vi "Handle Parameter Configuration File Change.vi"(8 "error in":errorcluster, 10 "new parameter configuration file path":path, 11 "Ballard MIL-STD-1553 custom device in":T1 format="%.0x") -> (0 "error out":errorcluster, 2 "parameters configuration file out":path, 3 "Ballard MIL-STD-1553 custom device out":T1 format="%.0x")   [LabVIEW 2020, in "Ballard MIL-STD-1553 System Explorer.lvlib" / "Implementation.lvlib" / "Refresh.lvlib"]
uses:
  Refresh.lvlib
  Scripting/Ballard MIL-STD-1553 Scripting.lvlib
  Import/MIL-STD 1553 Import.lvlib
  <vilib>/NI VeriStand/Custom Device API/Custom Device Item Ref.ctl
  <vilib>/NI VeriStand/Custom Device API/Custom Device API.lvlib
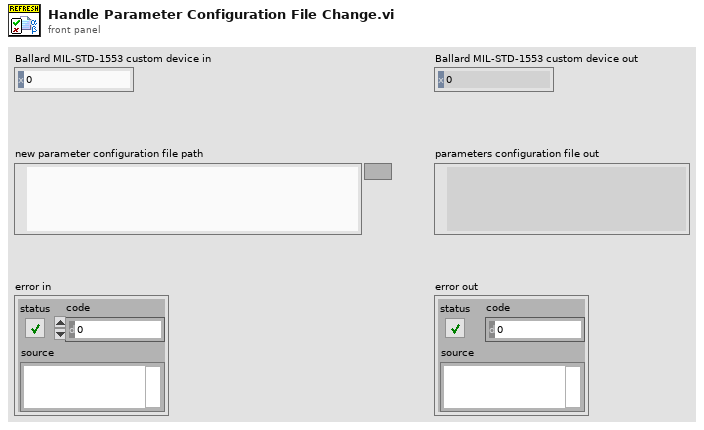
[diagram p1: front panel]
types:
  T1 = typedef "Custom Device API.lvlib/Custom Device Item Ref.ctl" = u64
  T2 = typedef "1553 Channel.ctl" = cluster{"HW channel":u16, "terminals":T3[], "messages":T5[], "acyclic frame names":string[]}
  T3 = typedef "Terminal Name and Address.ctl" = cluster{"name":string, "terminal address":T4}
  T4 = typedef "Address.ctl" = u16
  T5 = typedef "Message Definition.ctl" = cluster{"name":string, "message type":T6, "endpoint Rx":T7, "endpoint Tx":T7, "mode code":u16, "number of words":u16, "parameters":cluster{"name":string, "default value":dbl, "unit":string, "parameter definition":T8}[], "create timestamp channel":bool}
  T6 = typedef "Message Type.ctl" = string
  T7 = typedef "Terminal Endpoint.ctl" = cluster{"terminal address":T4, "subaddress":T4}
  T8 = typedef "Parameter Definition.ctl" = cluster{"start index":i32, "size (bits)":i32, "encoding":enum16{"BNR", "BCD", "Discrete"}, "signed":bool, "multiplier":dbl, "offset":dbl}
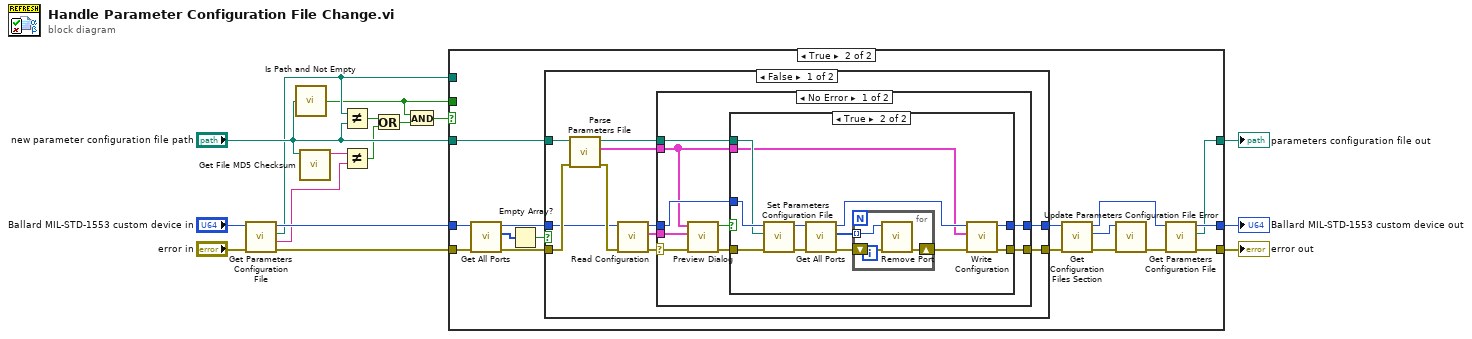
[diagram p0: block diagram]
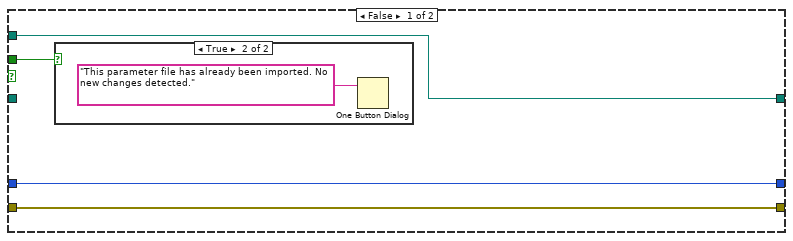
[diagram p2: hidden frame]
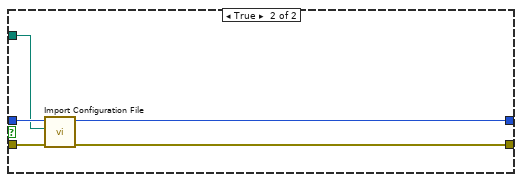
[diagram p6: hidden frame]
diagram:
  n1 = call "Get Parameters Configuration File.vi"("error in"="error in", "Ballard MIL-STD 1553 custom device in"="Ballard MIL-STD-1553 custom device in") -> ("error out"=w16:errorcluster, "MD5 checksum"=w8:string, "parameters configuration file"=w7:path, "Ballard MIL-STD 1553 custom device out"=w14:T1)  [unwired: 6 in]
  n2 = call <vilib>:"Is Path and Not Empty.vi"("path"="new parameter configuration file path") -> ("Is Path and Not Empty?"=w1:bool)  [unwired: 4 in]
  n3 = call "Get File MD5 Checksum.vi"("path"="new parameter configuration file path") -> ("MD5"=w4:string)  [unwired: 9 in, 1 out]
  n4 = Not Equal?(x=w7, y="new parameter configuration file path") -> (x != y?=w6:bool)
  n5 = Not Equal?(x=w4, y=w8) -> (x != y?=w5:bool)
  n6 = Or(x=w6, y=w5) -> (x .or. y?=w3:bool)
  n7 = And(x=w1, y=w3) -> (x .and. y?=w2:bool)
  n8 = case shown="True" w2 {
    tunnel: w16 -> [w19 w30]
    tunnel: w14 -> [w20 w31]
    tunnel: [w19 w25] -> w12
    tunnel: [w20 w23] -> w11
    tunnel: "new parameter configuration file path" -> [_ w32]
    tunnel: [w18 w22] -> w10
    tunnel: w7 -> [w18 _]
    tunnel: w1 -> [w17 _]
    frame False {
      n9 = case shown="True" w17 {
        frame False {
        }
        frame True {
          n10 = One Button Dialog(message="This parameter file has already been imported. No new changes detected.") -> ()  [unwired: 1 in, 1 out]
        }
      }
    }
    frame True {
      n11 = call "Get All Ports.vi"("error in"=w30, "Ballard MIL-STD 1553 custom device in"=w31) -> ("error out"=w29:errorcluster, "ports"=w27:T1[], "Ballard MIL-STD 1553 custom device out"=w28:T1)  [unwired: 7 in]
      n12 = Empty Array?(array=w27) -> (empty?=w26:bool)
      n13 = case shown="False" w26 {
        tunnel: [w40 w80] -> w35
        tunnel: [w38 w79] -> w34
        tunnel: w28 -> [w44 w78]
        tunnel: w29 -> [w46 w77]
        tunnel: w32 -> [w47 w76]
        frame False {
          n14 = call "Parse Parameters File.vi"("error in"=w46, "path to XML document"=w47) -> ("error out"=w45:errorcluster, "1553 channels"=w42:T2[], "path to XML document out"=w37:path)  [unwired: 7 in]
          n15 = call "Read Configuration.vi"("error in"=w45, "Ballard MIL-STD 1553 custom device in"=w44) -> ("error out"=w43:errorcluster, "1553 channels"=w41:T2[], "Ballard MIL-STD 1553 custom device out"=w39:T1)  [unwired: 7 in]
          n16 = case shown="No Error" w43 {
            selector: w43 -> [w55 w74]
            tunnel: w42 -> [w50 _]
            tunnel: w41 -> [w56 _]
            tunnel: [w49 w75] -> w40
            tunnel: w39 -> [w52 w75]
            tunnel: [w48 w74] -> w38
            tunnel: w37 -> [w51 _]
            frame No Error {
              n17 = call "Preview Dialog.vi"("error in"=w55, "current configuration"=w56, "new configuration"=w50) -> ("error out"=w53:errorcluster, "apply changes"=w54:bool)  [unwired: 7 in]
              n18 = case shown="True" w54 {
                tunnel: w53 -> [w57 w62]
                tunnel: w52 -> [w58 w64]
                tunnel: w51 -> [_ w63]
                tunnel: w50 -> [_ w61]
                tunnel: [w58 w60] -> w49
                tunnel: [w57 w59] -> w48
                frame False {
                }
                frame True {
                  n19 = call "Set Parameters Configuration File.vi"("error in"=w62, "parameters configuration file path"=w63, "Ballard MIL-STD 1553 custom device in"=w64) -> ("error out"=w69:errorcluster, "Ballard MIL-STD 1553 custom device out"=w70:T1)  [unwired: 7 in]
                  n20 = call "Get All Ports.vi"("error in"=w69, "Ballard MIL-STD 1553 custom device in"=w70) -> ("error out"=w68:errorcluster, "ports"=w65:T1[], "Ballard MIL-STD 1553 custom device out"=w66:T1)  [unwired: 7 in]
                  n21 = for {
                    shift-right: [w72] -> w67
                    shift-left: w68 -> [w73]
                    tunnel: w65 -> [w71] mode=indexing
                    n22 = call "Remove Port.vi"("error in"=w73, "port"=w71) -> ("error out"=w72:errorcluster)  [unwired: 9 in]
                  }
                  n23 = call "Write Configuration.vi"("error in"=w67, "1553 channels"=w61, "Ballard MIL-STD 1553 custom device in"=w66) -> ("error out"=w59:errorcluster, "Ballard MIL-STD 1553 custom device out"=w60:T1)  [unwired: 7 in]
                }
              }
            }
            frame Error {
            }
          }
        }
        frame True {
          n24 = call "Import Configuration File.vi"("error in"=w77, "parameters configuration file path"=w76, "Ballard MIL-STD 1553 custom device in"=w78) -> ("error out"=w79:errorcluster, "Ballard MIL-STD 1553 custom device out"=w80:T1)  [unwired: 7 in]
        }
      }
      n25 = call "Get Configuration Files Section.vi"("error in"=w34, "custom device in"=w35) -> ("error out"=w36:errorcluster, "configuration files section"=w33:T1, "custom device out"=w24:T1)  [unwired: 7 in]
      n26 = call "Update Parameters Configuration File Error.vi"("error in"=w36, "configuration files ref in"=w33) -> ("error out"=w25:errorcluster)  [unwired: 8 in, 1 out]
      n27 = call "Get Parameters Configuration File.vi"("error in"=w25, "Ballard MIL-STD 1553 custom device in"=w24) -> ("parameters configuration file"=w22:path, "Ballard MIL-STD 1553 custom device out"=w23:T1)  [unwired: 6 in, 2 out]
    }
  }
  "error out" <- w12
  "Ballard MIL-STD-1553 custom device out" <- w11
  "parameters configuration file out" <- w10
